vi "Error Loop.vi"(8 "error in":errorcluster) -> (0 "error out":errorcluster)   [LabVIEW 2019, in "TSC Error.lvlib"]
doc: "This loop runs in the top-level VI to handle Errors as they occur and will address them via Object Oriented code.\n\n<b>Note:</b> this should be a top-level loop running in parallel with the rest of the application\n\n<b>Code Developed By:</b>\nDaniel Coons\nTechnology Service Corporation\n1983 S Liberty Drive\nBloomington, IN 47403\nwww.tsc.com\\atcs"
uses:
  TSC Error.lvlib
  _Messages/Error/Error.lvclass
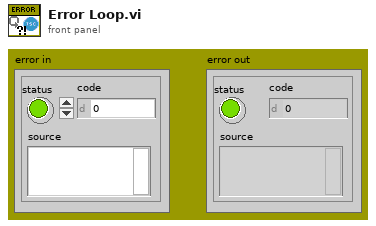
[diagram p1: front panel]
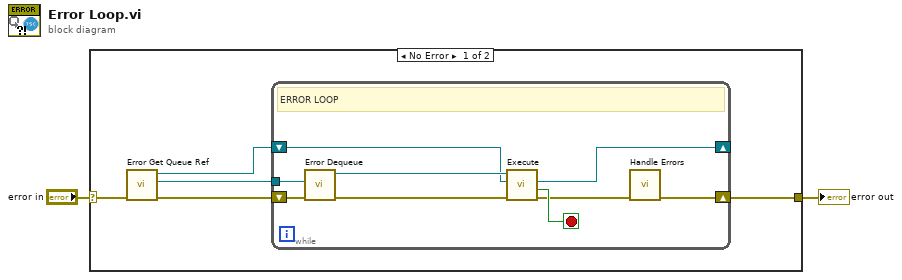
[diagram p0: block diagram]
diagram:
  n1 = case shown="No Error" "error in" {
    selector: "error in" -> [w5 w17]
    tunnel: [w7 w17] -> w1
    frame No Error {
      n2 = call "Error Get Queue Ref.vi"("error in (no error)"=w5) -> ("error out"=w6:errorcluster, "Error Queue out"=w4:refnum<queue>, "Error out"=w3:refnum<class "Error.lvclass">)  [unwired: 8 in]
      n3 = while {
        shift-right: [w11] -> w7
        shift-left: w6 -> [w15]
        tunnel: w4 -> [w8]
        shift-right: [w9] -> _
        shift-left: w3 -> [w10]
        stop <- w14 stop-if-true
        # "ERROR LOOP"
        n4 = call "Error Dequeue.vi"("error in"=w15, "Error Queue in"=w8) -> ("error out"=w16:errorcluster, "Error Message"=w13:refnum<class "Error.lvclass">)  [unwired: 8 in]
        n5 = call-dynamic "Execute.vi"("error in"=w16, "Shifted Error in"=w10, "Error in"=w13) -> ("error out"=w12:errorcluster, "STOP?"=w14:bool, "Shifted Error out"=w9:refnum<class "Error.lvclass">)  [unwired: 5 in, 1 out]
        n6 = call "Handle Errors.vi"("error in (no error)"=w12) -> ("error out"=w11:errorcluster)  [unwired: 10 in]
      }
    }
    frame Error {
    }
  }
  "error out" <- w1
